vi "BaselineCode_Template.vi"() -> ()   [LabVIEW 2026]
uses:
  <vilib>/numeric/Random Number (Range) U64.vi
  <vilib>/numeric/sub_Random U32.vi
panel:
  in  "Mode":enum32{"Simulated", "Hardware"}(radio)
  in  "Stop":bool
  in  "Buttons":bool[](array[boolean])
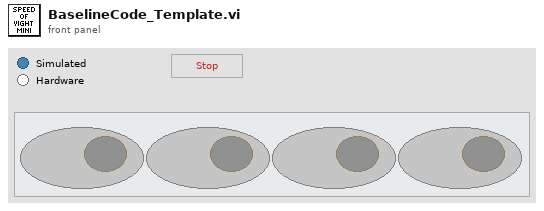
[diagram p1: front panel]
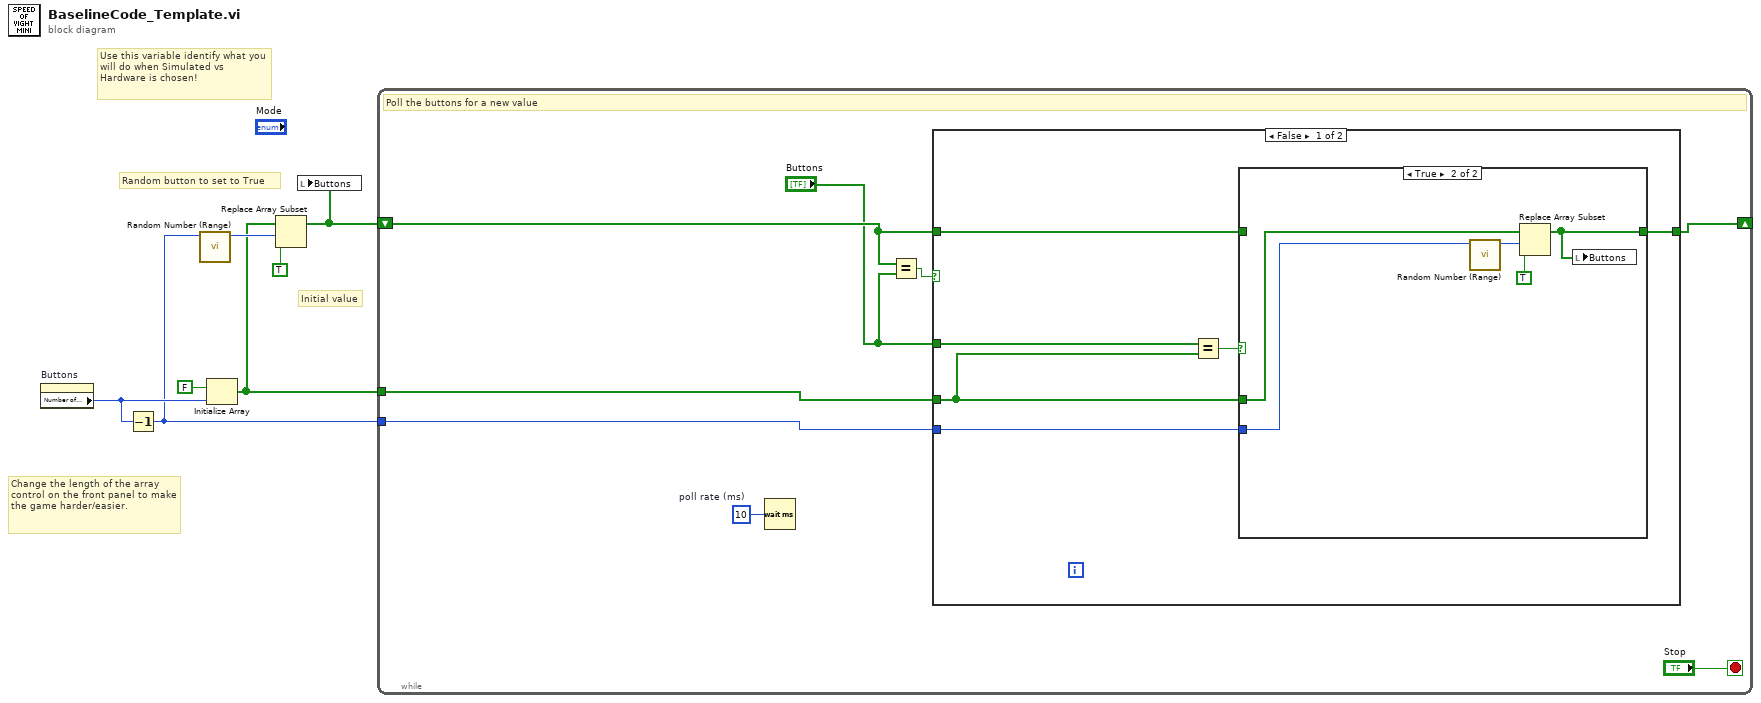
[diagram p0: block diagram]
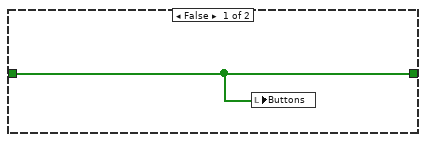
[diagram p2: hidden frame]
diagram:
  # "Use this variable identify what you will do when Simulated vs Hardware is chosen!"
  # "Random button to set to True"
  # "Initial value"
  # "Change the length of the array control on the front panel to make the game harder/easier."
  n1 = property on="Buttons" class="Arr (strict)"() -> ("Number of Columns"=w2:u32)  [unwired: 2 in, 2 out]
  n2 = Decrement(x=w2) -> (x-1=w1:u32)
  n3 = call-poly <vilib>:"Random Number (Range).vi"("upper bound (100)"=w1) -> ("number"=w6:u64)  [unwired: 10 in]
  n4 = Initialize Array(FALSE, w2) -> (w5:bool[])
  n5 = Replace Array Subset(array=w5, new element=TRUE ("new element/subarray"), index=w6) -> (w3:bool[])
  n6 = local write "Buttons"(w3) -> ()
  n7 = while {
    tunnel: w5 -> [w10]
    shift-right: [w11] -> _
    shift-left: w3 -> [w12]
    tunnel: w1 -> [w9]
    stop <- "Stop" stop-if-true
    w14 = u32 10  # poll rate (ms)
    # "Poll the buttons for a new value"
    n8 = Wait (ms)(milliseconds to wait=w14) -> ()  [unwired: 1 out]
    n9 = Equal?(x=w12, y="Buttons") -> (x = y?=w13:bool)
    n10 = case shown="False" w13 {
      tunnel: w12 -> [w16 w28]
      tunnel: [w18 w28] -> w11
      tunnel: w10 -> [w17 _]
      tunnel: "Buttons" -> [w21 _]
      tunnel: w9 -> [w19 _]
      frame False {
        # "Button value changed, see if they clicked the correct button."
        n11 = Equal?(x=w21, y=w17) -> (x = y?=w20:bool)
        n12 = case shown="True" w20 {
          tunnel: w19 -> [_ w24]
          tunnel: [w22 w23] -> w18
          tunnel: w17 -> [_ w25]
          tunnel: w16 -> [w22 _]
          frame False {
            # "Wrong button clicked. Decrement score and un-click button."
            n13 = local write "Buttons"(w22) -> ()
          }
          frame True {
            # "Correct button clicked, update score and set a new random value"
            n14 = call-poly <vilib>:"Random Number (Range).vi"("upper bound (100)"=w24) -> ("number"=w26:u64)  [unwired: 10 in]
            n15 = Replace Array Subset(array=w25, new element=TRUE ("new element/subarray"), index=w26) -> (w23:bool[])
            n16 = local write "Buttons"(w23) -> ()
          }
        }
      }
      frame True {
        # "Button value did not change"
      }
    }
  }
